vi "Update List of Connections.vi"(8 "error in (no error)":errorcluster, 10 "Item Names":string[][](array[string]), 11 "Server UI in":refnum<class "Server UI.lvclass">) -> (0 "error out":errorcluster, 3 "Server UI out":refnum<class "Server UI.lvclass">)   [LabVIEW 2015, in "Server UI.lvlib" / "Server UI.lvclass"]
uses:
  Server UI.lvclass
  Server UI.lvclass/Server UI.ctl
  <vilib>/ActorFramework/Actor/Actor.lvclass/Actor.ctl
  <vilib>/ActorFramework/Message Enqueuer/Message Enqueuer.lvclass/Message Enqueuer.ctl
  Read Connected Clients.vi
  <vilib>/ActorFramework/Message Enqueuer/Init from Existing Queue.vi
  <vilib>/ActorFramework/Message Enqueuer/Enqueue.vi
  <vilib>/ActorFramework/Message Priority Queue/Priority Enqueue.vi
  <vilib>/ActorFramework/Message Enqueuer/Message Enqueuer.lvclass
  <userlib>/Common Components/User Interface/Messages/Reset Controls Msg/Reset Controls Msg.lvclass
  Server UI Messages/Reset Measurement List Display Msg/Reset Measurement List Display Msg.lvclass
  <vilib>/ActorFramework/Actor/Actor.lvclass
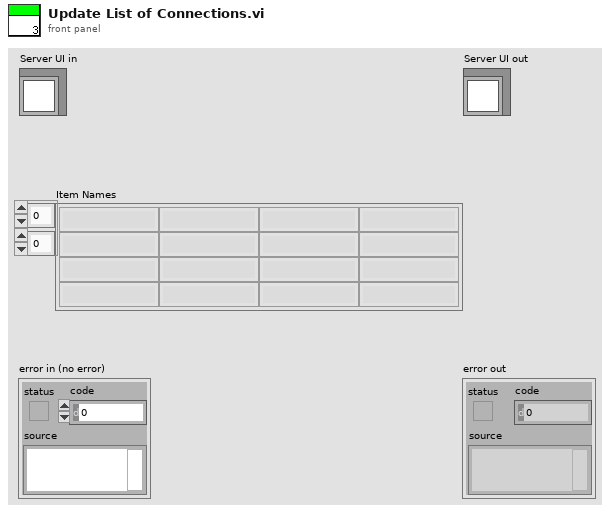
[diagram p1: front panel]
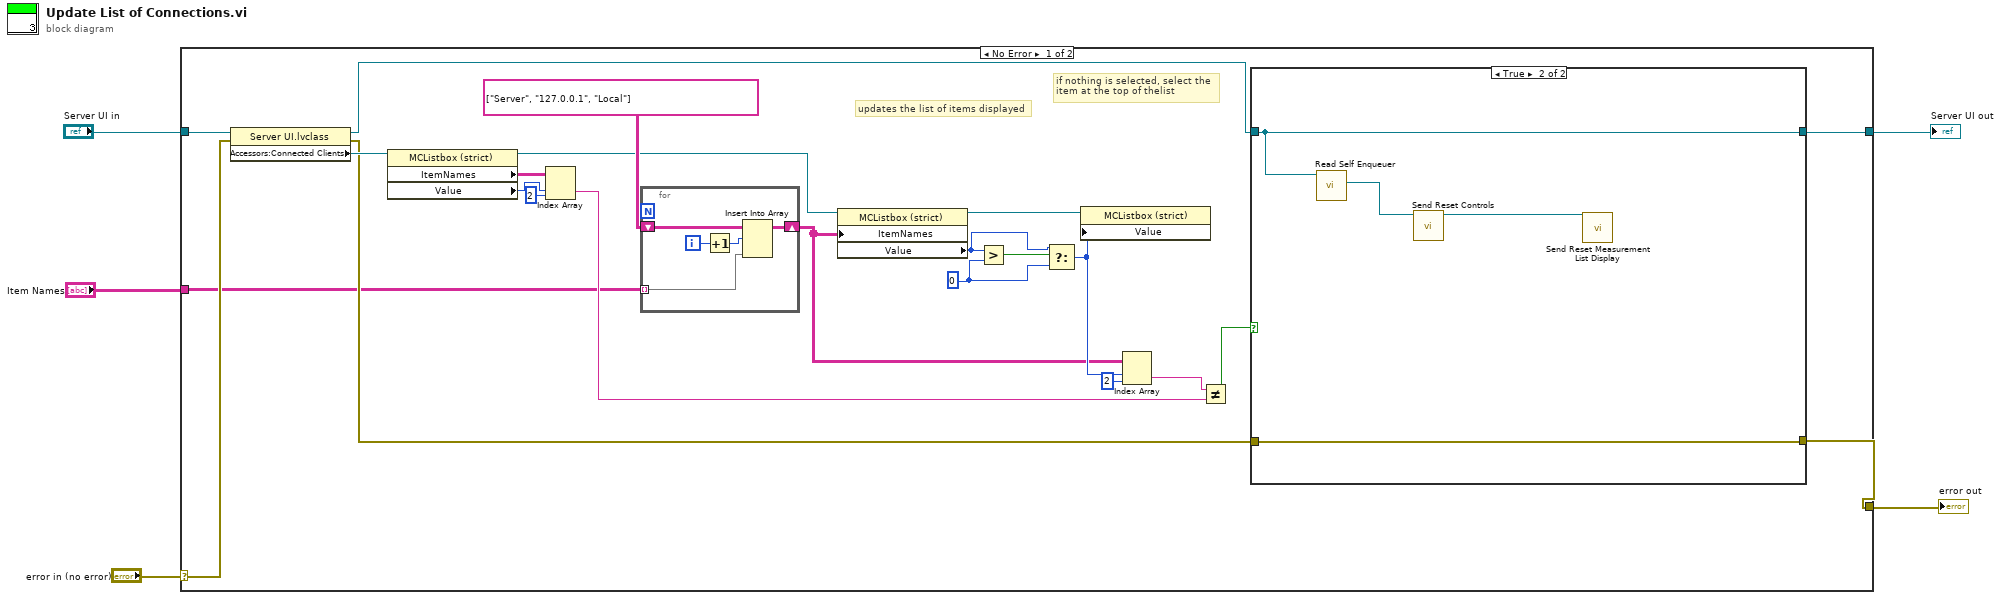
[diagram p0: block diagram]
diagram:
  n1 = case shown="No Error" "error in (no error)" {
    selector: "error in (no error)" -> [w12 w41]
    tunnel: [w11 w41] -> w4
    tunnel: [w15 w40] -> w2
    tunnel: "Server UI in" -> [w23 w40]
    tunnel: "Item Names" -> [w6 _]
    frame No Error {
      w24 = 0 ("y")
      # "updates the list of items displayed"
      # "if nothing is selected, select the \nitem at the top of thelist"
      n2 = property class="Server UI.lvclass"(reference=w23, error in=w12) -> (reference out=w22:refnum<class "Server UI.lvclass">, error out=w13:errorcluster, "Accessors:Connected Clients"=w21:refnum<vi>)
      n3 = property class="MCListbox (strict)"(reference=w21) -> (reference out=w10:refnum<vi>, "ItemNames"=w20:string[][], "Value"=w19:i32)  [unwired: 1 in, 1 out]
      n4 = Index Array(array=w20, index (row)=w19, index (col)=2 ("disabled index (col)")) -> (element=w16:string)
      n5 = for {
        shift-right: [w32] -> w9
        shift-left: string[][] [["Server", "127.0.0.1", "Local"]] ("element") -> [w33]
        tunnel: w6 -> [w29] mode=indexing
        i -> [w30]
        n6 = Increment(x=w30) -> (x+1=w31:i32)
        n7 = Insert Into Array(array=w33, index (row)=w31, new element=w29) -> (w32:string[][])  [unwired: 1 in]
      }
      n8 = property class="MCListbox (strict)"(reference=w10, "ItemNames"=w9) -> (reference out=w27:refnum<vi>, "Value"=w25:i32)  [unwired: 1 in, 1 out]
      n9 = Greater?(x=w25, y=w24) -> (0:w26:bool)
      n10 = Select(t=w25, s=w26, f=w24) -> (s? t:f=w18:i32)
      n11 = property class="MCListbox (strict)"(reference=w27, "Value"=w18) -> ()  [unwired: 1 in, 2 out]
      n12 = Index Array(array=w9, index (row)=w18, index (col)=2 ("disabled index (col)")) -> (element=w17:string)
      n13 = Not Equal?(x=w17, y=w16) -> (x != y?=w14:bool)
      n14 = case shown="True" w14 {
        tunnel: w22 -> [w35 w39]
        tunnel: [w35 w39] -> w15
        tunnel: w13 -> [w34 w38]
        tunnel: [w34 w38] -> w11
        frame False {
        }
        frame True {
          n15 = call <vilib>:"Read Self Enqueuer.vi"("Actor"=w39) -> ("Self Enqueuer"=w37:refnum<class "Message Enqueuer.lvclass">)  [unwired: 10 in]
          n16 = call <userlib>:"Send Reset Controls.vi"("Message Enqueuer"=w37) -> ("Message Enqueuer out"=w36:refnum<class "Message Enqueuer.lvclass">)  [unwired: 9 in, 1 out]
          n17 = call "Send Reset Measurement List Display.vi"("Message Enqueuer"=w36) -> ()  [unwired: 9 in, 2 out]
        }
      }
    }
    frame Error {
    }
  }
  "error out" <- w4
  "Server UI out" <- w2
